vi "Stop API.vi"(8 "Error In":errorcluster) -> (0 "Error Out":errorcluster)   [LabVIEW 2017, in "Auto cycle.lvlib"]
uses:
  Auto cycle.lvlib
  Events/Events.lvlib
  Controls/Commands [enum].ctl
  Controls/Command Data [cluster].ctl
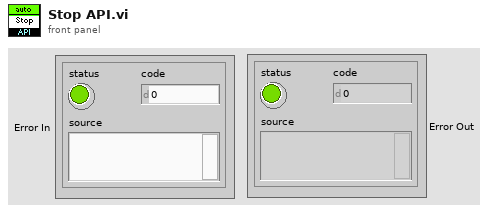
[diagram p1: front panel]
types:
  T1 = typedef "Auto cycle.lvlib/Command Data [cluster].ctl" = cluster{"Command":T2, "Data":variant}
  T2 = typedef "Auto cycle.lvlib/Commands [enum].ctl" = enum16{"Start", "Stop", "Send config"}
  T3 = typedef "Events.lvlib/Refs [cluster].ctl" = cluster{"Exit":refnum<user-event>, "Controller":refnum<user-event>, "System Error":refnum<user-event>, "UI":refnum<user-event>, "Example Module":refnum<user-event>, "Shutter":refnum<user-event>, "Monochromator":refnum<user-event>, "DAQ":refnum<user-event>, "Example Module 2":refnum<user-event>}
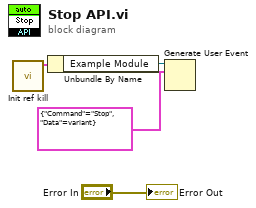
[diagram p0: block diagram]
diagram:
  n1 = call "Init ref kill.vi"() -> ("Messages"=w4:T3)  [unwired: 10 in, 1 out]
  n2 = Unbundle By Name(w4) -> ("Example Module"=w3:refnum<user-event>)
  n3 = Generate User Event(user event=w3, event data cluster=T1 {"Command"=enum."Stop", "Data"=variant} ("event data")) -> ()  [unwired: 2 in, 2 out]
  "Error Out" <- "Error In"
